vi "Get Parameter Value by Name.vi"(0 "Parameter Array":string[](array[string]), 7 "Parameter Name":string) -> (4 "Parameter Array Out":string[](array[string]), 8 "Found?":bool, 10 "Flattened Value":string)   [LabVIEW 2014]
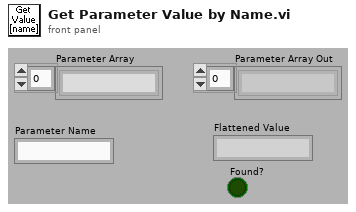
[diagram p1: front panel]
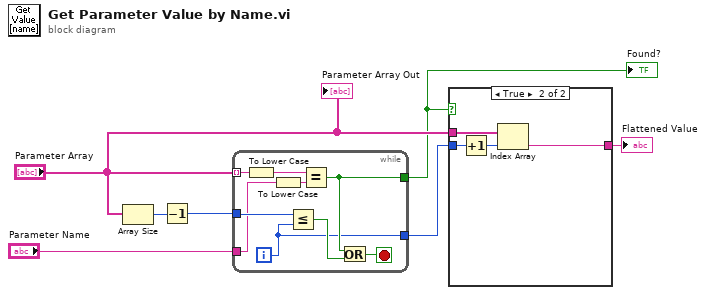
[diagram p0: block diagram]
diagram:
  n1 = Array Size(array="Parameter Array") -> (size(s)=w1:i32)
  n2 = Decrement(x=w1) -> (x-1=w2:i32)
  n3 = while {
    tunnel: "Parameter Array" -> [w15] mode=indexing
    tunnel: w2 -> [w16]
    tunnel: "Parameter Name" -> [w14]
    tunnel: [w9] -> w4
    tunnel: [w8] -> w5
    i -> [w8]
    stop <- w13 stop-if-true
    n4 = To Lower Case(string=w15) -> (all lower case string=w11:string)
    n5 = To Lower Case(string=w14) -> (all lower case string=w10:string)
    n6 = Less Or Equal?(x=w16, y=w8) -> (x <= y?=w12:bool)
    n7 = Equal?(x=w11, y=w10) -> (x = y?=w9:bool)
    n8 = Or(x=w9, y=w12) -> (x .or. y?=w13:bool)
  }
  "Found?" <- w4
  n9 = case shown="True" w4 {
    tunnel: w5 -> [_ w20]
    tunnel: "Parameter Array" -> [_ w19]
    tunnel: [_ w18] -> w7
    frame False {
    }
    frame True {
      n10 = Increment(x=w20) -> (x+1=w17:i32)
      n11 = Index Array(array=w19, index=w17) -> (element=w18:string)
    }
  }
  "Flattened Value" <- w7
  "Parameter Array Out" <- "Parameter Array"
